vi "DISPLAY  tdms file v1.vi"() -> ()   [LabVIEW 2013]
panel:
  out "error out":errorcluster
  in  "file path":path
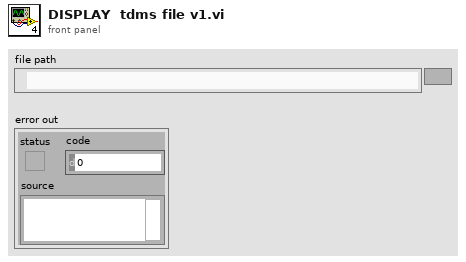
[diagram p1: front panel]
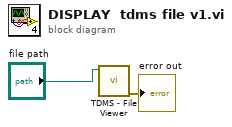
[diagram p0: block diagram]
diagram:
  n1 = call <vilib>:"TDMS - File Viewer.vi"("file path"="file path") -> ("error out"=→"error out":errorcluster)  [unwired: 5 in, 1 out]
